vi "COD主界面（列队使用）.vi"() -> (8 "多列列表框":i32(listbox))   [LabVIEW 2016, in "斯坦道CODMn.lvlib"]
uses:
  <vilib>/Utility/miscctls.llb/LVPointTypeDef.ctl
  <vilib>/Plasmionique/MB Master/MB_Master_Serial/MB_Master_Serial.lvclass
  F:/Program Files/National Instruments/LabVIEW 2016/vi.lib/Plasmionique/MB Master/MB_Master/MB_Master.lvclass
  <vilib>/Plasmionique/MB Master/MB Master.lvlib
  <vilib>/ptbypt/NI_PtbyPt.lvlib
  PLC/PLC.lvlib
panel:
  out "启动选择 3":u16(ring) items=["COD水样测量", "COD标样核查", "COD零点核查", "COD加标回收", "COD平行样", "COD校零", "COD校标", ""]
  out "加热":bool
  out "搅拌":bool
  out "进硫酸":bool
  out "进草酸钠":bool
  out "进高锰酸钾":bool
  out "进加标回收样":bool
  out "进质控样":bool
  out "进标液":bool
  out "进蒸馏水":bool
  out "进水样":bool
  in  "定时启动":bool
  out "设置值":dbl
  out "系统时间":timestamp
  in  "时间校准":bool
  out "仪器时间":timestamp
  in  "修正系数 2":dbl
  in  "浓度 2":dbl
  in  "温度":dbl
  out "秒":u16
  out "分":u16
  in  "data in":T1
  out "数值":i32
  out "报警簇":T2
  out "读取参数":u16[](array[numeric])
  out "循环次数":i32
  out "DATABASE":u16[](array[numeric])
  out "Registers":u16[](array[numeric])
  in  "枚举":enum16{"读取数据", "写入数据", "读取写入DATABASE", "读取参数"}(ring)
  in  "Slave ID":u8=1
  in  "Serial Config":T3={"baud rate (bps)"=115200, "stop bits"=10, "parity"=0, "flow control"=0, "timeout"=1000, "retries"=1} {"stop bits" items=["1.0"=10, "1.5"=15, "2.0"=20]; "flow control" items=["None", "XON/XOFF", "RTS/CTS", "XON/XOFF & RTS/CTS", "DTR/DSR", "XON/XOFF & DTR/DSR"]; "parity" items=["None", "Odd", "Even", "Mark", "Space"]}
  out "COD浓度（mg/L)":dbl
  out "table 输入":string
  out "columns":string[](array[string])
  in  "保存":bool
  out "data":T4
  in  "温度 2":dbl
  in  "恒温时间":dbl
  in  "浓度":dbl
  in  "修正系数":dbl
  in  "基本量程":enum16{"10mL", "20mL"}(ring)
  in  "水样":dbl
  in  "蒸馏水":dbl
  in  "标液":dbl
  in  "质控样":dbl
  in  "加标回收":dbl
  in  "草酸钠":dbl
  in  "高锰酸钾":dbl
  in  "硫酸":dbl
  in  "关闭":bool
  in  "零点泵计量数 2":dbl
  in  "标度泵计量数 2":dbl
  in  "标样浓度 2":dbl
  out "进样管":dbl
  out "高锰酸钾":dbl
  out "草酸钠":dbl
  out "硫酸":dbl
  out "标度滴定值":dbl
  out "零点滴定值":dbl
  in  "启动":bool
  in  "故障清除":bool
  out "排液故障":bool
  out "进水样超量程":bool
  out "模式（受控）":u16
  out "ORP显示":dbl
  out "温度":dbl
  out "标样核查标记":bool
  out "平行样测量":bool
  out "加标回收测量":bool
  out "质控样测量":bool
  out "待机":bool
  out "校标错误":bool
  out "校零错误":bool
  out "测量错误":bool
  out "草酸钠报警":bool
  out "高锰酸钾报警":bool
  out "加热故障":bool
  out "温控器故障":bool
  out "ORP故障":bool
  out "排液标记":bool
  out "故障标记":bool
  out "校标标记":bool
  out "校零标记":bool
  out "通讯状态":bool
  out "水样测量":bool
  in  "参数配置":bool
  in  "VISA resource name":refnum<visa-resource-name>="COM3" caption="VISA资源名称"
  in  "停止":bool
  in  "单步启动":bool
  # "测量时间："
  # "水样~加标回收"
  # "mV"
  # "℃"
  # "注：遇到加热故障和排液故障时仪器不能正常启动，\n必须排查故障并点击报警清除按钮方可运行。"
  # "基本参数设置"
  # "泵计量参数设置"
  # "校零校标结果"
  # "加热恒温温度（℃）："
  # "水样："
  # "高锰酸钾："
  # "校零结果："
  # "校零滴定值："
  # "恒温时间（分钟）："
  # "蒸馏水："
  # "草酸钠："
  # "校标结果："
  # "标度滴定值："
  # "零点泵计量值："
  # "标准液浓度（mg/L）："
  # "标液："
  # "硫酸："
  # "标样浓度："
  # "标度泵计量值："
  # "修正系数："
  # "质控样："
  # "加标回收样："
  # "基本量程（20mL可选）："
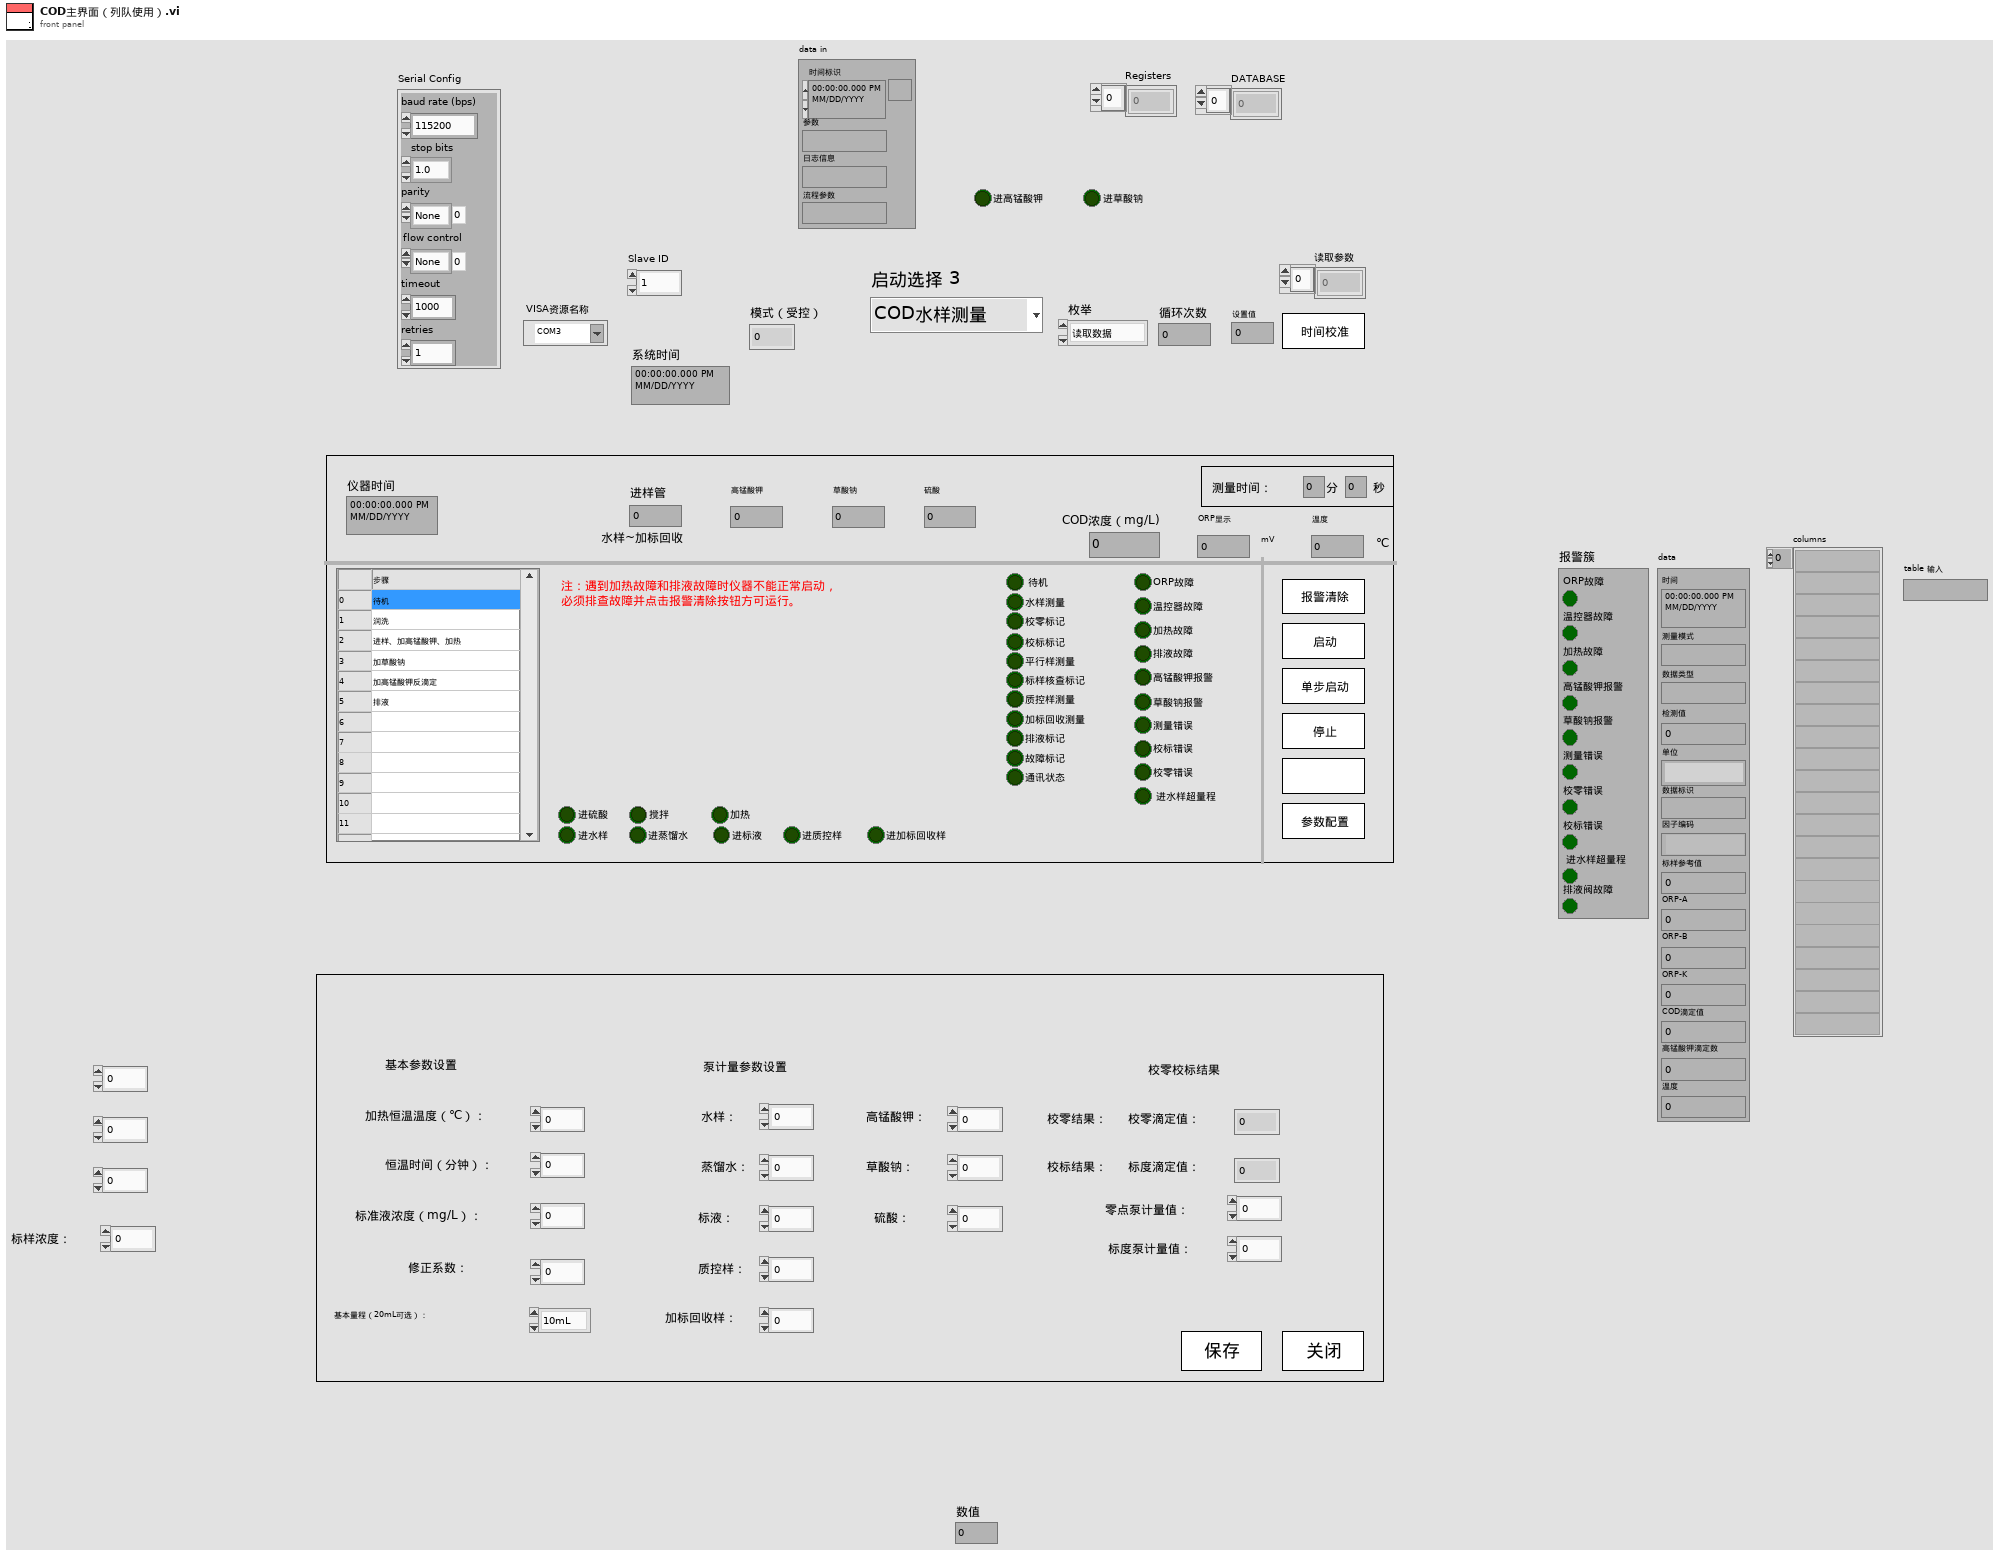
[diagram p1: front panel]
types:
  T1 = cluster{"时间标识":timestamp, "参数":string, "日志信息":string, "流程参数":string}
  T2 = cluster{"ORP故障":bool, "温控器故障":bool, "加热故障":bool, "高锰酸钾报警":bool, "草酸钠报警":bool, "测量错误":bool, "校零错误":bool, "校标错误":bool, " 进水样超量程":bool, "排液阀故障":bool}
  T3 = cluster{"baud rate (bps)":u32, "stop bits":u16, "parity":u16, "flow control":u16, "timeout":u32, "retries":i32}
  T4 = cluster{"时间":timestamp, "测量模式":string, "数据类型":string, "检测值":sgl, "单位":string, "数据标识":string, "因子编码":string, "标样参考值":sgl, "ORP-A":sgl, "ORP-B":sgl, "ORP-K":sgl, "COD滴定值":sgl, "高锰酸钾滴定数":sgl, "温度":sgl}
  T5 = cluster{"starting address":u16, "number of holding registers":u16}
  T6 = typedef "LVPointTypeDef.ctl" = cluster{"Horizontal":i16, "Vertical":i16}
  T7 = cluster{"测量模式":enum16{"水样测量", "标样核查", "零点核查", "加标回收", "平行样", "校零", "校标"}}
  T8 = cluster{"时间标识":timestamp, "设备":string, "日志信息":string}
  T9 = cluster{"时间标识":timestamp, "设备":string, "日志信息":string, "流程参数":string}
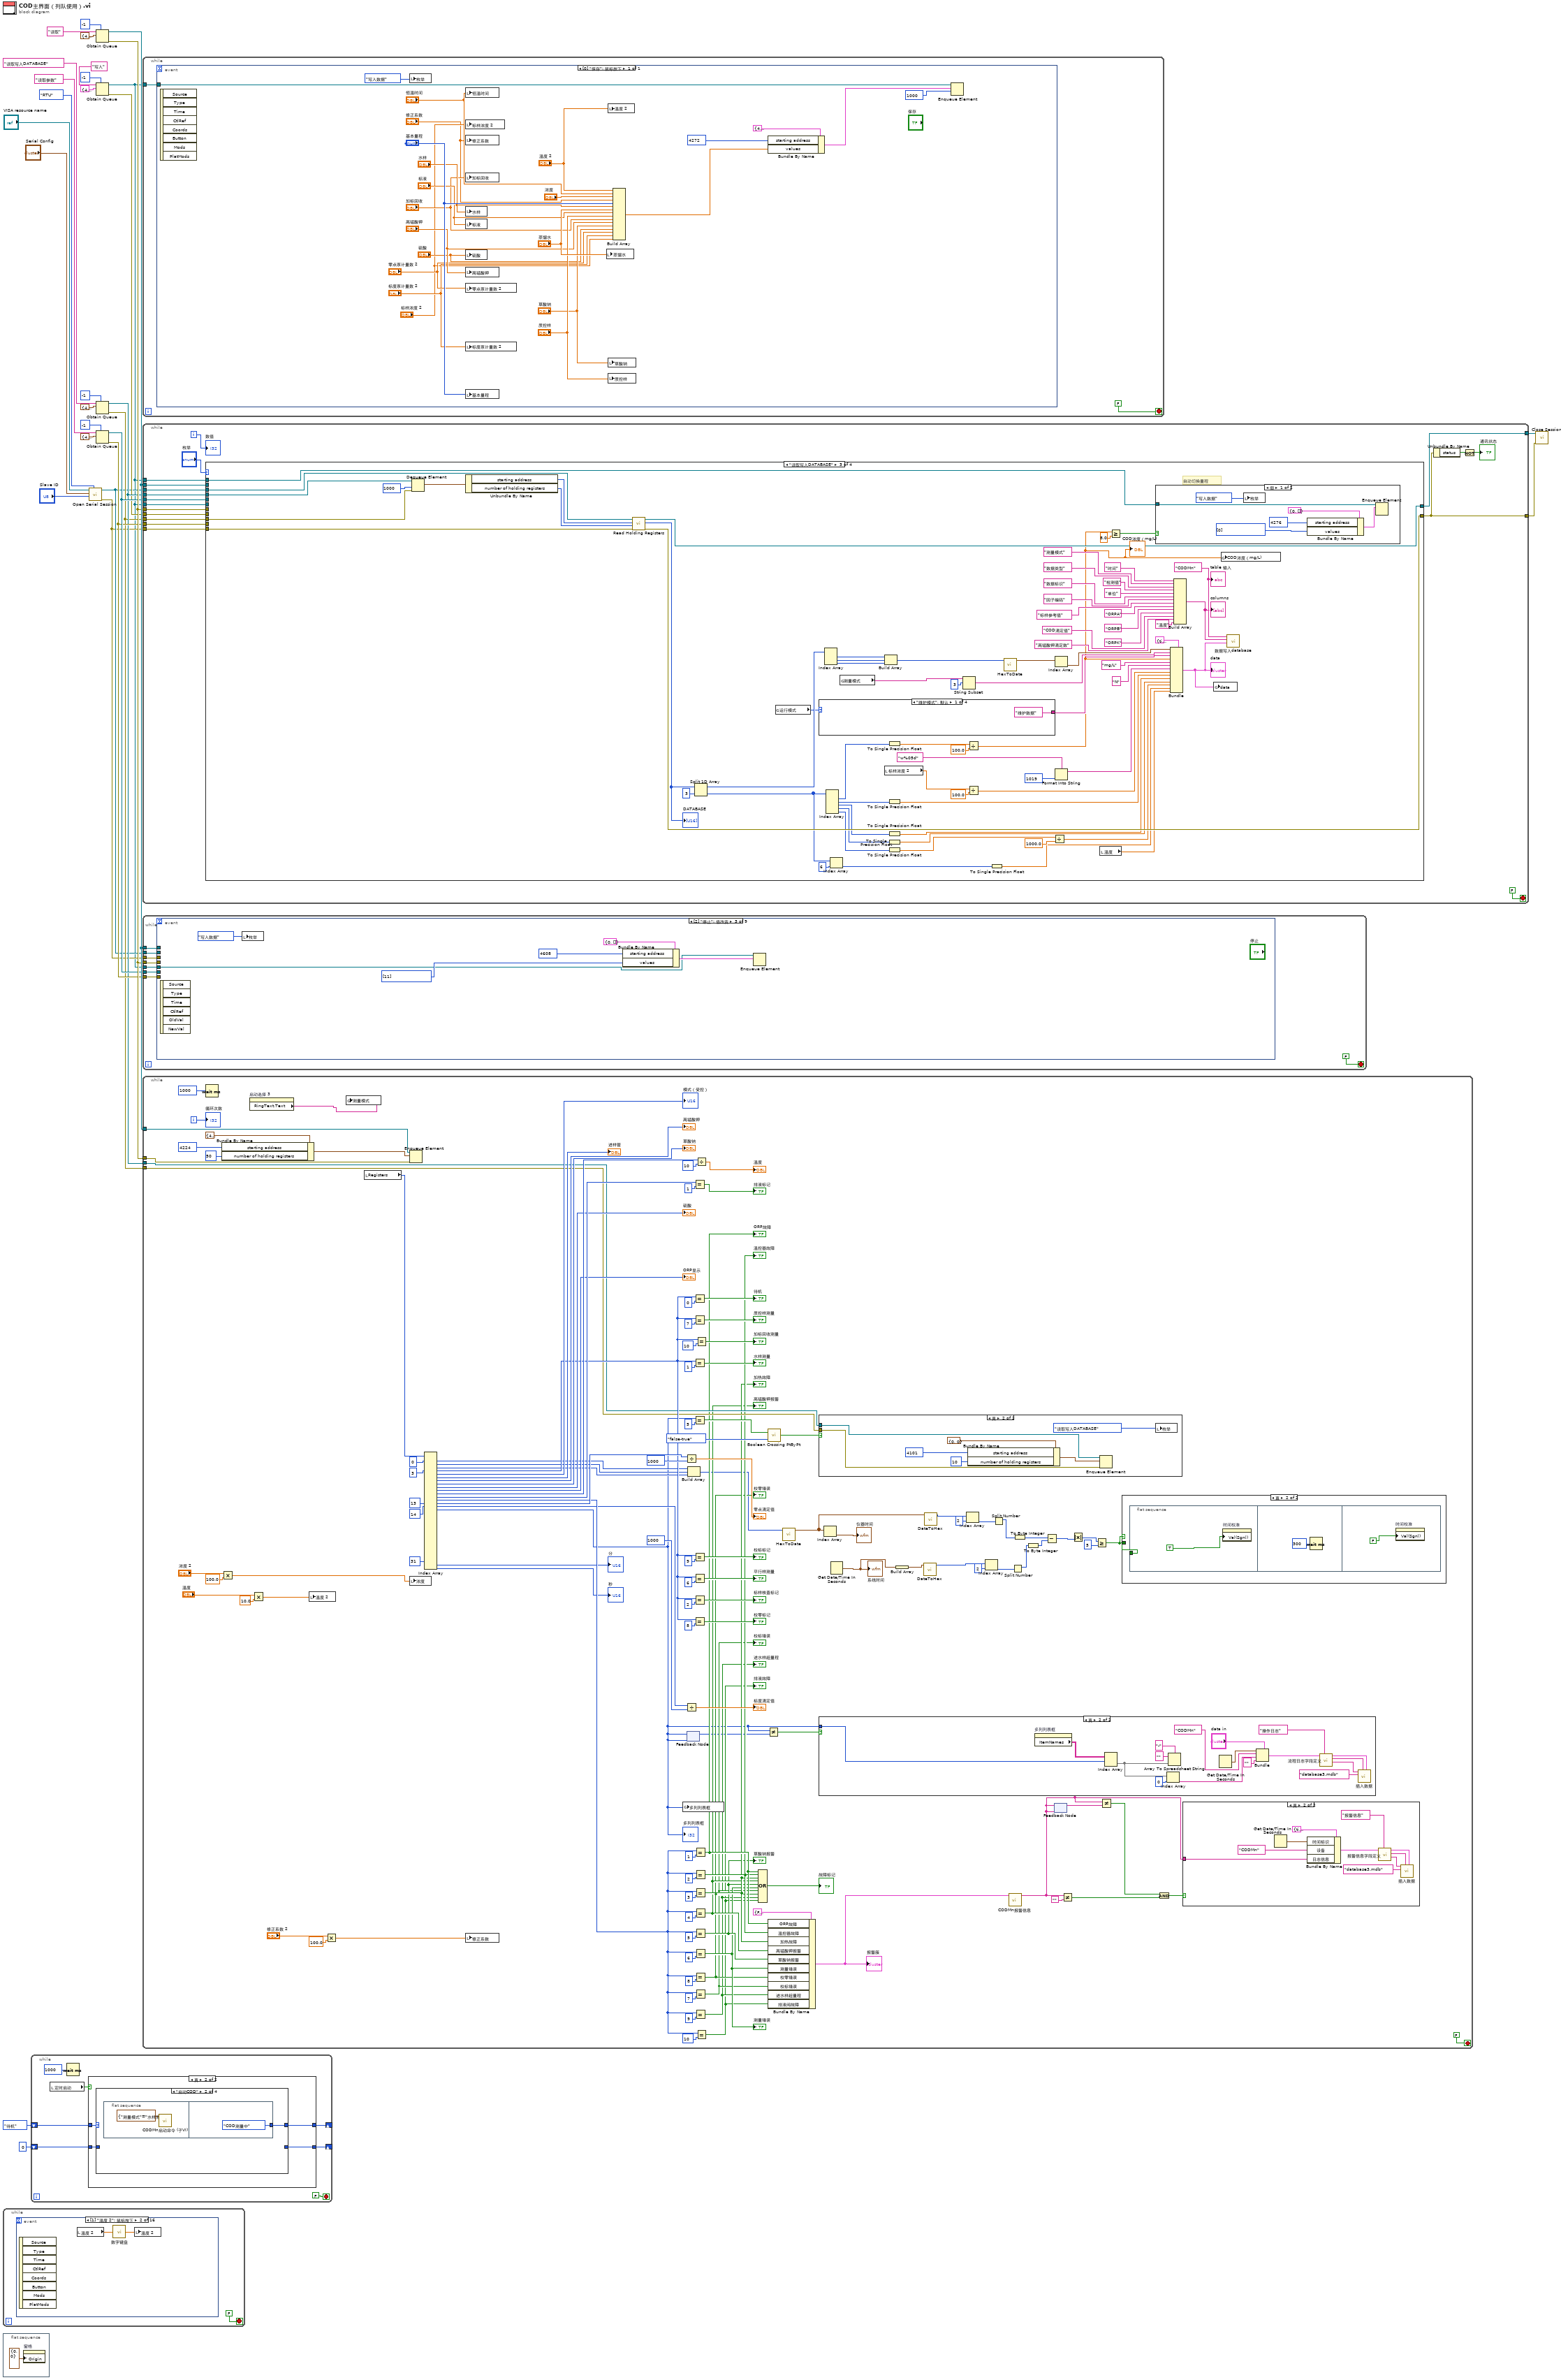
[diagram p0: block diagram]
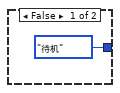
[diagram p2: hidden frame]
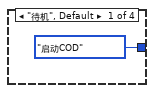
[diagram p3: hidden frame]
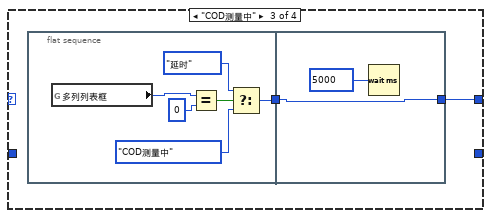
[diagram p4: hidden frame]
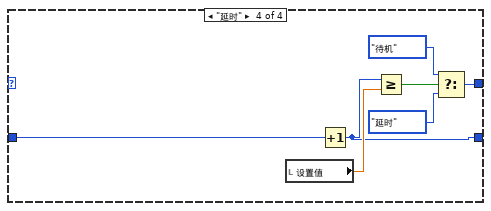
[diagram p5: hidden frame]
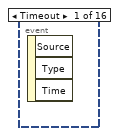
[diagram p10: hidden frame]
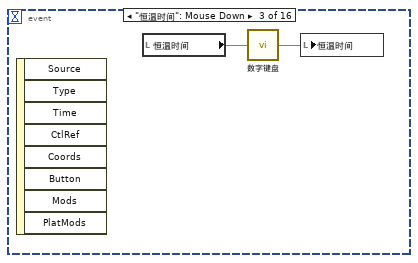
[diagram p11: hidden frame]
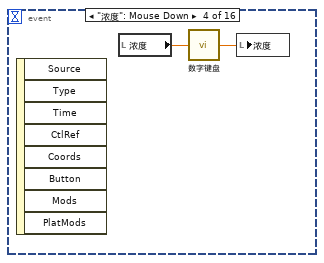
[diagram p12: hidden frame]
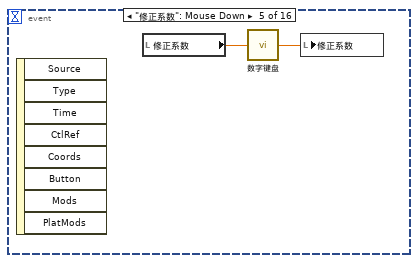
[diagram p13: hidden frame]
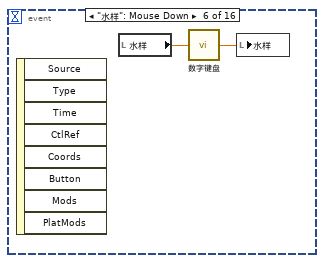
[diagram p14: hidden frame]
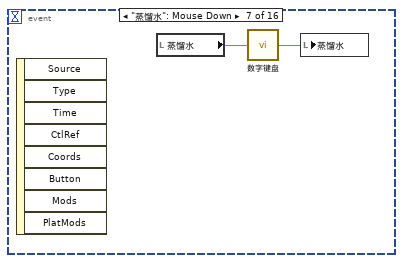
[diagram p15: hidden frame]
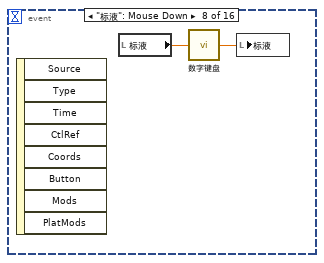
[diagram p16: hidden frame]
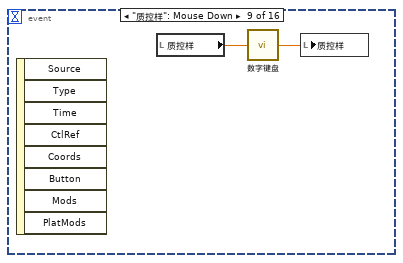
[diagram p17: hidden frame]
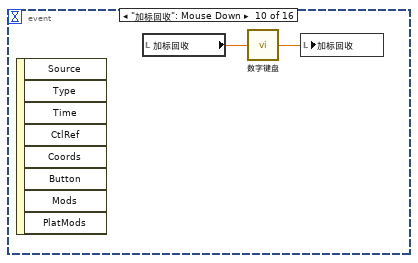
[diagram p18: hidden frame]
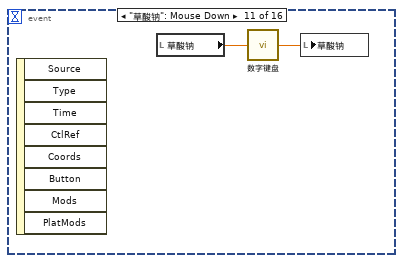
[diagram p19: hidden frame]
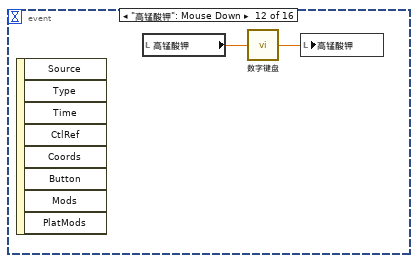
[diagram p20: hidden frame]
diagram:
  n1 = while {
    stop <- FALSE stop-if-true
    n2 = event shown="[1] \"温度 2\": 鼠标按下" {
      selector: _ -> [_ _ _ _ _ _ _ _ _ _ _ _ _ _ _ _]
      dyn-events: _ -> [_ _ _ _ _ _ _ _ _ _ _ _ _ _ _ _]
      timeout: _ -> [_ _ _ _ _ _ _ _ _ _ _ _ _ _ _ _]
      event Timeout {
        n3 = event-data() -> ()  [unwired: 1 in, 3 out]
      }
      event "温度 2": Mouse Down {
        n4 = event-data() -> ()  [unwired: 1 in, 8 out]
        n5 = local read "温度 2"() -> (w32:dbl)
        n6 = call "数字键盘.vi"("OldNumber"=w32) -> ("NewNumber"=w33:sgl)
        n7 = local write "温度 2"(w33) -> ()
      }
      event "恒温时间": Mouse Down {
        n8 = event-data() -> ()  [unwired: 1 in, 8 out]
        n9 = local read "恒温时间"() -> (w34:dbl)
        n10 = call "数字键盘.vi"("OldNumber"=w34) -> ("NewNumber"=w35:sgl)
        n11 = local write "恒温时间"(w35) -> ()
      }
      event "浓度": Mouse Down {
        n12 = event-data() -> ()  [unwired: 1 in, 8 out]
        n13 = local read "浓度"() -> (w36:dbl)
        n14 = call "数字键盘.vi"("OldNumber"=w36) -> ("NewNumber"=w37:sgl)
        n15 = local write "浓度"(w37) -> ()
      }
      event "修正系数": Mouse Down {
        n16 = event-data() -> ()  [unwired: 1 in, 8 out]
        n17 = local read "修正系数"() -> (w38:dbl)
        n18 = call "数字键盘.vi"("OldNumber"=w38) -> ("NewNumber"=w39:sgl)
        n19 = local write "修正系数"(w39) -> ()
      }
      event "水样": Mouse Down {
        n20 = event-data() -> ()  [unwired: 1 in, 8 out]
        n21 = local read "水样"() -> (w40:dbl)
        n22 = call "数字键盘.vi"("OldNumber"=w40) -> ("NewNumber"=w41:sgl)
        n23 = local write "水样"(w41) -> ()
      }
      event "蒸馏水": Mouse Down {
        n24 = event-data() -> ()  [unwired: 1 in, 8 out]
        n25 = local read "蒸馏水"() -> (w42:dbl)
        n26 = call "数字键盘.vi"("OldNumber"=w42) -> ("NewNumber"=w43:sgl)
        n27 = local write "蒸馏水"(w43) -> ()
      }
      event "标液": Mouse Down {
        n28 = event-data() -> ()  [unwired: 1 in, 8 out]
        n29 = local read "标液"() -> (w44:dbl)
        n30 = call "数字键盘.vi"("OldNumber"=w44) -> ("NewNumber"=w45:sgl)
        n31 = local write "标液"(w45) -> ()
      }
      event "质控样": Mouse Down {
        n32 = event-data() -> ()  [unwired: 1 in, 8 out]
        n33 = local read "质控样"() -> (w46:dbl)
        n34 = call "数字键盘.vi"("OldNumber"=w46) -> ("NewNumber"=w47:sgl)
        n35 = local write "质控样"(w47) -> ()
      }
      event "加标回收": Mouse Down {
        n36 = event-data() -> ()  [unwired: 1 in, 8 out]
        n37 = local read "加标回收"() -> (w48:dbl)
        n38 = call "数字键盘.vi"("OldNumber"=w48) -> ("NewNumber"=w49:sgl)
        n39 = local write "加标回收"(w49) -> ()
      }
      event "草酸钠": Mouse Down {
        n40 = event-data() -> ()  [unwired: 1 in, 8 out]
        n41 = local read "草酸钠"() -> (w50:dbl)
        n42 = call "数字键盘.vi"("OldNumber"=w50) -> ("NewNumber"=w51:sgl)
        n43 = local write "草酸钠"(w51) -> ()
      }
      event "高锰酸钾": Mouse Down {
        n44 = event-data() -> ()  [unwired: 1 in, 8 out]
        n45 = local read "高锰酸钾"() -> (w52:dbl)
        n46 = call "数字键盘.vi"("OldNumber"=w52) -> ("NewNumber"=w53:sgl)
        n47 = local write "高锰酸钾"(w53) -> ()
      }
      event "硫酸": Mouse Down {
        n48 = event-data() -> ()  [unwired: 1 in, 8 out]
        n49 = local read "硫酸"() -> (w54:dbl)
        n50 = call "数字键盘.vi"("OldNumber"=w54) -> ("NewNumber"=w55:sgl)
        n51 = local write "硫酸"(w55) -> ()
      }
      event "零点泵计量数 2": Mouse Down {
        n52 = event-data() -> ()  [unwired: 1 in, 8 out]
        n53 = local read "零点泵计量数 2"() -> (w56:dbl)
        n54 = call "数字键盘.vi"("OldNumber"=w56) -> ("NewNumber"=w57:sgl)
        n55 = local write "零点泵计量数 2"(w57) -> ()
      }
      event "标度泵计量数 2": Mouse Down {
        n56 = event-data() -> ()  [unwired: 1 in, 8 out]
        n57 = local read "标度泵计量数 2"() -> (w58:dbl)
        n58 = call "数字键盘.vi"("OldNumber"=w58) -> ("NewNumber"=w59:sgl)
        n59 = local write "标度泵计量数 2"(w59) -> ()
      }
      event "标样浓度 2": Mouse Down {
        n60 = event-data() -> ()  [unwired: 1 in, 8 out]
        n61 = local read "标样浓度 2"() -> (w60:dbl)
        n62 = call "数字键盘.vi"("OldNumber"=w60) -> ("NewNumber"=w61:sgl)
        n63 = local write "标样浓度 2"(w61) -> ()
      }
    }
  }
  n64 = flat-sequence {
    frame #0 {
      n65 = property on="窗格" class="Pane"("Origin"=T6 {"Horizontal"=0, "Vertical"=0} ("原点")) -> ()  [unwired: 2 in, 2 out]
    }
  }
  n66 = while {
    shift-right: [w64] -> _
    shift-left: enum16{"待机", "启动COD", "COD测量中", "延时"}."待机" -> [w66]
    shift-right: [w63] -> _
    shift-left: 0 -> [w65]
    stop <- FALSE stop-if-true
    n67 = local read "定时启动"() -> (w68:bool)
    n68 = Wait (ms)(milliseconds to wait=u32 1000 ("等待时间（毫秒）")) -> ()  [unwired: 1 out]
    n69 = case shown="真" w68 {
      tunnel: w66 -> [_ w74]
      tunnel: w65 -> [_ w73]
      tunnel: [enum16{"待机", "启动COD", "COD测量中", "延时"}."待机" w72] -> w64
      tunnel: [_ w71] -> w63
      frame False {
      }
      frame True {
        n70 = case shown="\"启动COD\"" w74 {
          tunnel: w73 -> [_ _ _ w95]
          tunnel: [enum16{"待机", "启动COD", "COD测量中", "延时"}."启动COD" w76 w80 w89] -> w72
          tunnel: [_ _ _ w92] -> w71
          frame "待机", Default {
          }
          frame "启动COD" {
            n71 = flat-sequence {
              tunnel: [enum16{"待机", "启动COD", "COD测量中", "延时"}."COD测量中"] -> w76
              frame #0 {
                n72 = call "CODMn启动命令 (子VI).vi"("启动测量模式"=T7 {"测量模式"=enum."水样测量"}) -> ()  [unwired: 11 in]
              }
              frame #1 {
              }
            }
          }
          frame "COD测量中" {
            n73 = flat-sequence {
              tunnel: [w81] -> w79
              tunnel: [w88] -> w80
              tunnel: w79 -> [w88]
              frame #0 {
                n74 = global read "运行时序全局变量.vi" "多列列表框"() -> (w86:i32)
                n75 = Equal?(x=w86, y=0) -> (x = y?=w84:bool)
                n76 = Select(t=enum16{"待机", "启动COD", "COD测量中", "延时"}."延时", s=w84, f=enum16{"待机", "启动COD", "COD测量中", "延时"}."COD测量中") -> (s? t:f=w81:enum16{"待机", "启动COD", "COD测量中", "延时"})
              }
              frame #1 {
                n77 = Wait (ms)(milliseconds to wait=u32 5000 ("等待时间（毫秒）")) -> ()  [unwired: 1 out]
              }
            }
          }
          frame "延时" {
            n78 = local read "设置值"() -> (w94:dbl)
            n79 = Increment(x=w95) -> (x+1=w92:i32)
            n80 = Greater Or Equal?(x=w92, y=w94) -> (x >= y?=w93:bool)
            n81 = Select(t=enum16{"待机", "启动COD", "COD测量中", "延时"}."待机", s=w93, f=enum16{"待机", "启动COD", "COD测量中", "延时"}."延时") -> (s? t:f=w89:enum16{"待机", "启动COD", "COD测量中", "延时"})
          }
        }
      }
    }
  }
  n82 = call <vilib>:"Open Serial Session.vi"("Mode (RTU)"=enum16{"RTU", "ASCII"}."RTU", "Slave ID"="Slave ID", "Serial Config"="Serial Config", "VISA Resource"="VISA resource name") -> ("Error out"=w4:errorcluster, "MB_Serial session"=w5:refnum<class "MB_Master_Serial.lvclass">)  [unwired: 6 in]
  n83 = Obtain Queue(max queue size (-1, unlimited)=-1 ("队列最大值（-1，无限）"), name (unnamed)="读取" ("名称（未命名）"), element data type=T5 {"starting address"=4224, "number of holding registers"=16}) -> (queue out=w20:refnum<queue>, error out=w19:errorcluster)  [unwired: 2 in, 1 out]
  n84 = Obtain Queue(max queue size (-1, unlimited)=-1 ("队列最大值（-1，无限）"), name (unnamed)="写入" ("名称（未命名）"), element data type=cluster{"starting address":u16, "values":u16[]} {"starting address"=4272, "values"=[]}) -> (queue out=w1:refnum<queue>, error out=w6:errorcluster)  [unwired: 2 in, 1 out]
  n85 = Obtain Queue(max queue size (-1, unlimited)=-1 ("队列最大值（-1，无限）"), name (unnamed)="读取写入DATABASE" ("名称（未命名）"), element data type=T5 {"starting address"=4224, "number of holding registers"=16}) -> (queue out=w8:refnum<queue>, error out=w7:errorcluster)  [unwired: 2 in, 1 out]
  n86 = Obtain Queue(max queue size (-1, unlimited)=-1 ("队列最大值（-1，无限）"), name (unnamed)="读取参数" ("名称（未命名）"), element data type=T5 {"starting address"=4224, "number of holding registers"=16}) -> (queue out=w13:refnum<queue>, error out=w12:errorcluster)  [unwired: 2 in, 1 out]
  n87 = while {
    tunnel: w1 -> [w97]
    stop <- FALSE stop-if-true
    n88 = event shown="[0] \"保存\": 鼠标按下" {
      selector: _ -> [_]
      dyn-events: _ -> [_]
      timeout: _ -> [_]
      tunnel: w97 -> [w107]
      event "保存": Mouse Down {
        n89 = event-data() -> ()  [unwired: 1 in, 8 out]
        n90 = local write "枚举"(enum16{"读取数据", "写入数据", "读取写入DATABASE", "读取参数"}."写入数据" ("枚举")) -> ()
        n91 = local write "恒温时间"("恒温时间") -> ()
        n92 = local write "标样浓度 2"("标样浓度 2") -> ()
        n93 = local write "修正系数"("修正系数") -> ()
        n94 = local write "加标回收"("加标回收") -> ()
        n95 = local write "水样"("水样") -> ()
        n96 = local write "标液"("标液") -> ()
        n97 = local write "硫酸"("硫酸") -> ()
        n98 = local write "高锰酸钾"("高锰酸钾") -> ()
        n99 = local write "零点泵计量数 2"("零点泵计量数 2") -> ()
        n100 = local write "标度泵计量数 2"("标度泵计量数 2") -> ()
        n101 = local write "基本量程"("基本量程") -> ()
        n102 = local write "蒸馏水"("蒸馏水") -> ()
        n103 = local write "温度 2"("温度 2") -> ()
        n104 = local write "草酸钠"("草酸钠") -> ()
        n105 = local write "质控样"("质控样") -> ()
        n106 = Build Array("温度 2", "恒温时间", "浓度", "修正系数", "基本量程", "水样", "蒸馏水", "标液", "质控样", "加标回收", "高锰酸钾", "草酸钠", "硫酸", "零点泵计量数 2", "标度泵计量数 2", "标样浓度 2") -> (w105:dbl[])
        n107 = Bundle By Name(cluster=cluster{"starting address":u16, "values":u16[]} {"starting address"=4272, "values"=[]}, "starting address"=u16 4272, "values"=w105) -> (w103:cluster{"starting address":u16, "values":u16[]})
        n108 = Enqueue Element(queue=w107, element=w103, timeout in ms (-1)=1000 ("超时毫秒(-1)")) -> ()  [unwired: 1 in, 3 out]
      }
    }
  }
  n109 = while {
    tunnel: w5 -> [w138]
    tunnel: w4 -> [w137]
    tunnel: w1 -> [w136]
    tunnel: w20 -> [w135]
    tunnel: w19 -> [w134]
    tunnel: [w124] -> w18
    tunnel: [w133] -> w17
    tunnel: w13 -> [w131]
    tunnel: w12 -> [w130]
    tunnel: w8 -> [w129]
    tunnel: w7 -> [w128]
    tunnel: w6 -> [w127]
    tunnel: w1 -> [w121]
    i -> [w123]
    stop <- FALSE stop-if-true
    n110 = case shown="\"读取写入DATABASE\"" "枚举" {
      tunnel: w138 -> [w174 w182 w262 w311]
      tunnel: w137 -> [w173 w178 w261 w310]
      tunnel: w136 -> [_ w181 _ _]
      tunnel: [w147 w180 w264 w313] -> w133
      tunnel: [w146 w179 w263 w312] -> w124
      tunnel: w135 -> [w171 _ _ _]
      tunnel: w134 -> [w167 _ _ _]
      tunnel: w131 -> [_ _ _ w309]
      tunnel: w130 -> [_ _ _ w308]
      tunnel: w129 -> [_ _ w260 _]
      tunnel: w128 -> [_ _ w259 _]
      tunnel: w127 -> [_ w177 _ _]
      tunnel: w121 -> [_ _ w199 _]
      frame "读取数据", Default {
        n111 = Dequeue Element(queue=w171, timeout in ms (-1)=1000 ("超时毫秒(-1)"), error in (no error)=w167) -> (element=w170:T5)  [unwired: 3 out]
        n112 = Unbundle By Name(w170) -> ("starting address"=w169:u16, "number of holding registers"=w168:u16)
        n113 = call <vilib>:"Read Holding Registers.vi"("error in (no error)"=w173, "quantity"=w168, "starting address"=w169, "MB session in"=w174) -> ("error out"=w162:errorcluster, "Registers"=→"Registers":u16[], "MB session out"=w165:refnum<class "MB_Master_Serial.lvclass">)  [unwired: 5 in]
        n114 = call <vilib>:"Read Coils.vi"("error in (no error)"=w162, "quantity"=u16 8, "starting address"=u16 140, "MB session in"=w165) -> ("error out"=w152:errorcluster, "Coils"=w161:bool[], "MB session out"=w153:refnum<class "MB_Master_Serial.lvclass">)  [unwired: 5 in]
        n115 = Index Array(array=w161) -> (element #1=→"进水样":bool, element #2=→"进蒸馏水":bool, element #3=→"进标液":bool, element #4=→"进质控样":bool, element #5=→"进加标回收样":bool, element #6=→"进高锰酸钾":bool, element #7=→"进草酸钠":bool, element #8=→"进硫酸":bool)  [unwired: 9 in, 1 out]
        n116 = call <vilib>:"Read Coils.vi"("error in (no error)"=w152, "quantity"=u16 1, "starting address"=u16 137, "MB session in"=w153) -> ("error out"=w148:errorcluster, "Coils"=w140:bool[], "MB session out"=w149:refnum<class "MB_Master_Serial.lvclass">)  [unwired: 5 in]
        n117 = Index Array(array=w140) -> (element=→"搅拌":bool)  [unwired: 1 in]
        n118 = call <vilib>:"Read Coils.vi"("error in (no error)"=w148, "quantity"=u16 1, "starting address"=u16 400, "MB session in"=w149) -> ("error out"=w146:errorcluster, "Coils"=w143:bool[], "MB session out"=w147:refnum<class "MB_Master_Serial.lvclass">)  [unwired: 5 in]
        n119 = Index Array(array=w143) -> (element=→"加热":bool)  [unwired: 1 in]
      }
      frame "写入数据" {
        n120 = flat-sequence {
          tunnel: w182 -> [w192]
          tunnel: w181 -> [w191]
          tunnel: w178 -> [w185]
          tunnel: w177 -> [w184]
          tunnel: [w187] -> w176
          tunnel: [w186] -> w175
          tunnel: [w194] -> w179
          tunnel: [w195] -> w180
          tunnel: w176 -> [w195]
          tunnel: w175 -> [w194]
          frame #0 {
            n121 = Dequeue Element(queue=w191, error in (no error)=w184) -> (queue out=w183:refnum<queue>, element=w190:cluster{"starting address":u16, "values":u16[]})  [unwired: 1 in, 2 out]
            n122 = Flush Queue(queue=w183) -> ()  [unwired: 1 in, 3 out]
            n123 = Unbundle By Name(w190) -> ("starting address"=w189:u16, "values"=w188:u16[])
            n124 = call <vilib>:"Write Multiple Registers.vi"("error in (no error)"=w185, "values"=w188, "starting address"=w189, "MB session in"=w192) -> ("error out"=w186:errorcluster, "MB session out"=w187:refnum<class "MB_Master_Serial.lvclass">)  [unwired: 6 in]
          }
          frame #1 {
            n125 = local write "枚举"(enum16{"读取数据", "写入数据", "读取写入DATABASE", "读取参数"}."读取数据" ("枚举")) -> ()
          }
        }
      }
      frame "读取写入DATABASE" {
        w227 = "CODMn" ("table")
        # "自动切换量程"
        n126 = Dequeue Element(queue=w260, timeout in ms (-1)=1000 ("超时毫秒(-1)"), error in (no error)=w259) -> (element=w267:T5)  [unwired: 3 out]
        n127 = Unbundle By Name(w267) -> ("starting address"=w266:u16, "number of holding registers"=w265:u16)
        n128 = call <vilib>:"Read Holding Registers.vi"("error in (no error)"=w261, "quantity"=w265, "starting address"=w266, "MB session in"=w262) -> ("error out"=w263:errorcluster, "Registers"=w223:u16[], "MB session out"=w264:refnum<class "MB_Master_Serial.lvclass">)  [unwired: 5 in]
        "DATABASE" <- w223
        n129 = Split 1D Array(array=w223, index=3 ("索引")) -> (first subarray=w257:u16[], second subarray=w245:u16[])
        n130 = global read "系统变量.vi" "运行模式"() -> (w206:enum16{"维护模式", "常规模式", "应急模式", "质控模式"})
        n131 = case shown="\"维护模式\", 默认" w206 {
          tunnel: ["维护数据" ("单位") "常规数据" ("单位") "常规数据" ("单位") "常规数据" ("单位")] -> w205
          frame "维护模式", Default {
          }
          frame "常规模式" {
          }
          frame "应急模式" {
          }
          frame "质控模式" {
          }
        }
        n132 = Index Array(array=w257) -> (element #1=w255:u16, element #2=w254:u16, element #3=w253:u16)  [unwired: 3 in]
        n133 = Index Array(array=w245) -> (element #1=w250:u16, element #2=w249:u16, element #3=w248:u16, element #4=w247:u16, element #5=w246:u16)  [unwired: 5 in]
        n134 = Index Array(array=w245, index=6 ("索引")) -> (element=w243:u16)
        n135 = global read "COD测量模式全局.vi" "测量模式"() -> (w196:string)
        n136 = Build Array(w255, w254, w253) -> (w252:u16[])
        n137 = local read "标样浓度 2"() -> (w221:dbl)
        n138 = To Single Precision Float(number=w250) -> (single precision float=w242:sgl)
        n139 = To Single Precision Float(number=w249) -> (single precision float=w211:sgl)
        n140 = To Single Precision Float(number=w248) -> (single precision float=w212:sgl)
        n141 = To Single Precision Float(number=w247) -> (single precision float=w213:sgl)
        n142 = To Single Precision Float(number=w246) -> (single precision float=w239:sgl)
        n143 = String Subset(string=w196, offset (0)=3 ("偏移量(0)")) -> (substring=w202:string)  [unwired: 1 in]
        n144 = Divide(x=w242, y=sgl 100.0) -> (x/y=w197:sgl)
        "COD浓度（mg/L)" <- w197
        n145 = Divide(x=w221, y=100.0) -> (x/y=w210:dbl)
        n146 = To Single Precision Float(number=w243) -> (single precision float=w215:sgl)
        n147 = call "HexToDate.vi"("数组"=w252) -> ("DATE"=w256:timestamp[])  [unwired: 10 in]
        n148 = Divide(x=w239, y=sgl 1000.0) -> (x/y=w214:sgl)
        n149 = Index Array(array=w256) -> (element=w251:timestamp)  [unwired: 1 in]
        n150 = Format Into String(format string="w%05d" ("格式字符串"), u32 1019 ("因子编码")) -> (resulting string=w209:string)  [unwired: 2 in, 1 out]
        n151 = local read "温度"() -> (w204:dbl)
        n152 = Greater Or Equal?(x=w197, y=sgl 8.0) -> (x >= y?=w200:bool)
        n153 = case shown="假" w200 {
          tunnel: w199 -> [w268 w277]
          frame False {
            n154 = local write "枚举"(enum16{"读取数据", "写入数据", "读取写入DATABASE", "读取参数"}."写入数据" ("枚举")) -> ()
            n155 = Bundle By Name(cluster=cluster{"starting address":u16, "values":u16[]} {"starting address"=0, "values"=[]}, "starting address"=u16 4276, "values"=u16[] [0]) -> (w271:cluster{"starting address":u16, "values":u16[]})
            n156 = Enqueue Element(queue=w268, element=w271) -> ()  [unwired: 2 in, 3 out]
          }
          frame True {
            n157 = local write "枚举"(enum16{"读取数据", "写入数据", "读取写入DATABASE", "读取参数"}."写入数据" ("枚举")) -> ()
            n158 = Bundle By Name(cluster=cluster{"starting address":u16, "values":u16[]} {"starting address"=0, "values"=[]}, "starting address"=u16 4276, "values"=u16[] [1]) -> (w278:cluster{"starting address":u16, "values":u16[]})
            n159 = Enqueue Element(queue=w277, element=w278) -> ()  [unwired: 2 in, 3 out]
          }
        }
        n160 = Bundle(cluster=T4 {"时间"=timestamp(0 s since 1904-01-01), "测量模式"="", "数据类型"="", "检测值"=0.0, "单位"="", "数据标识"="", "因子编码"="", "标样参考值"=0.0, "ORP-A"=0.0, "ORP-B"=0.0, "ORP-K"=0.0, "COD滴定值"=0.0, "高锰酸钾滴定数"=0.0, "温度"=0.0} ("data"), "时间"=w251, "测量模式"=w202, "数据类型"=w205, "检测值"=w197, "单位"="mg/L", "数据标识"="N", "因子编码"=w209, "标样参考值"=w210, "ORP-A"=w211, "ORP-B"=w212, "ORP-K"=w213, "COD滴定值"=w214, "高锰酸钾滴定数"=w215, "温度"=w204) -> (w198:T4)
        "data" <- w198
        n161 = Build Array("时间", "测量模式", "数据类型", "检测值", "单位", "数据标识", "因子编码", "标样参考值", "ORPA", "ORPB", "ORPK", "COD滴定值", "高锰酸钾滴定数", "温度") -> (w226:string[])
        "columns" <- w226
        n162 = global write "COD读取DATA全局.vi" "data"(w198) -> ()
        n163 = global write "COD浓度全局变量.vi" "COD浓度（mg/L)"(w197) -> ()
        n164 = call "数据写入database.vi"("data"=w198, "columns"=w226, "table"=w227) -> ()  [unwired: 9 in]
        "table 输入" <- w227
      }
      frame "读取参数" {
        n165 = Dequeue Element(queue=w309, timeout in ms (-1)=1000 ("超时毫秒(-1)"), error in (no error)=w308) -> (element=w317:T5)  [unwired: 3 out]
        n166 = local write "枚举"(enum16{"读取数据", "写入数据", "读取写入DATABASE", "读取参数"}."读取数据" ("枚举")) -> ()
        n167 = Unbundle By Name(w317) -> ("starting address"=w316:u16, "number of holding registers"=w315:u16)
        n168 = call <vilib>:"Read Holding Registers.vi"("error in (no error)"=w310, "quantity"=w315, "starting address"=w316, "MB session in"=w311) -> ("error out"=w312:errorcluster, "Registers"=w294:u16[], "MB session out"=w313:refnum<class "MB_Master_Serial.lvclass">)  [unwired: 5 in]
        "读取参数" <- w294
        n169 = Index Array(array=w294) -> (element #1=w287:u16, element #2=w307:u16, element #3=w306:u16, element #4=w285:u16, element #5=w305:u16, element #6=w304:u16, element #7=w303:u16, element #8=w302:u16, element #9=w301:u16, element #10=w300:u16, element #11=w299:u16, element #12=w298:u16, element #13=w297:u16, element #14=w296:u16, element #15=w295:u16, element #16=w292:u16)  [unwired: 16 in]
        n170 = local write "浓度"(w306) -> ()
        n171 = local write "水样"(w304) -> ()
        n172 = local write "硫酸"(w297) -> ()
        n173 = local write "标液"(w302) -> ()
        n174 = local write "恒温时间"(w307) -> ()
        n175 = local write "基本量程"(w305) -> ()
        n176 = local write "加标回收"(w300) -> ()
        n177 = local write "高锰酸钾"(w299) -> ()
        n178 = local write "草酸钠"(w298) -> ()
        n179 = local write "零点泵计量数 2"(w296) -> ()
        n180 = local write "标度泵计量数 2"(w295) -> ()
        n181 = local write "蒸馏水"(w303) -> ()
        n182 = local write "质控样"(w301) -> ()
        n183 = Divide(x=w287, y=u16 10) -> (x/y=w288:dbl)
        n184 = Divide(x=w285, y=u16 100) -> (x/y=w284:dbl)
        n185 = Divide(x=w292, y=u16 100) -> (x/y=w291:dbl)
        n186 = local write "温度"(w288) -> ()
        n187 = local write "修正系数 2"(w284) -> ()
        n188 = local write "浓度 2"(w291) -> ()
      }
    }
    n189 = Unbundle By Name(w124) -> ("status"=w125:bool)
    n190 = Not(x=w125) -> (.not. x?=→"通讯状态":bool)
    "数值" <- w123
  }
  n191 = while {
    tunnel: w20 -> [w325]
    tunnel: w19 -> [w324]
    tunnel: w1 -> [w323]
    tunnel: w13 -> [w322]
    tunnel: w12 -> [w321]
    tunnel: w5 -> [w319]
    tunnel: w4 -> [w318]
    stop <- FALSE stop-if-true
    n192 = event shown="[2] \"停止\": 值改变" {
      selector: _ -> [_ _ _ _ _ _ _ _ _]
      dyn-events: _ -> [_ _ _ _ _ _ _ _ _]
      timeout: _ -> [_ _ _ _ _ _ _ _ _]
      tunnel: w325 -> [_ _ _ _ _ _ _ _ _]
      tunnel: w324 -> [_ _ _ _ _ _ _ _ _]
      tunnel: w323 -> [w332 w366 w387 _ _ _ w405 w419 _]
      tunnel: w322 -> [_ _ _ w393 _ _ _ _ _]
      tunnel: w321 -> [_ _ _ w392 _ _ _ _ _]
      tunnel: w319 -> [_ _ _ _ _ w404 _ _ _]
      tunnel: w318 -> [_ _ _ _ _ w403 _ _ _]
      event "单步启动": Mouse Down {
        n193 = event-data() -> ()  [unwired: 1 in, 8 out]
        n194 = call "单步启动选择对话框.vi"() -> ("启动选择 2"=w335:u16)  [unwired: 10 in, 1 out]
        n195 = case shown="0" w335 {
          tunnel: [u16 4610 ("address") u16 4610 ("address") u16 4610 ("address") u16 4610 ("address") u16 4610 ("address") u16 4610 ("address") u16 4610 ("address") u16 4610 ("address") u16 4610 ("address") u16 4610 ("address") u16 4610 ("address") u16 4610 ("address")] -> w331
          tunnel: [u16 1 ("address") u16 2 ("address") u16 3 ("address") u16 4 ("address") u16 5 ("address") u16 6 ("address") u16 7 ("address") u16 8 ("address") u16 9 ("holding register value") u16 10 ("holding register value") u16 11 ("holding register value") u16 0 ("address")] -> w328
          frame 0 {
          }
          frame 1 {
          }
          frame 2 {
          }
          frame 3 {
          }
          frame 4 {
          }
          frame 5 {
          }
          frame 6 {
          }
          frame 7 {
          }
          frame 8 {
          }
          frame 9 {
          }
          frame 10 {
          }
          frame 11, Default {
          }
        }
        n196 = local write "枚举"(enum16{"读取数据", "写入数据", "读取写入DATABASE", "读取参数"}."写入数据" ("枚举")) -> ()
        n197 = Insert Into Array(array=u16[] [] ("values"), index=0 ("索引"), new element=w328) -> (w327:u16[])
        n198 = Bundle By Name(cluster=cluster{"starting address":u16, "values":u16[]} {"starting address"=0, "values"=[]}, "starting address"=w331, "values"=w327) -> (w333:cluster{"starting address":u16, "values":u16[]})
        n199 = Enqueue Element(queue=w332, element=w333) -> ()  [unwired: 2 in, 3 out]
      }
      event "启动": Mouse Down {
        n200 = event-data() -> ()  [unwired: 1 in, 8 out]
        n201 = call "启动测量模式选择对话框.vi"() -> ("启动选择 3"=w369:u16)  [unwired: 11 in]
        "启动选择 3" <- w369
        n202 = case shown="7, 默认" w369 {
          tunnel: [u16 4608 ("address") u16 4608 ("address") u16 4608 ("address") u16 4608 ("address") u16 4608 ("address") u16 4608 ("address") u16 4608 ("address") u16 4608 ("address")] -> w365
          tunnel: [u16 1 ("address") u16 2 ("address") u16 3 ("address") u16 7 ("address") u16 6 ("address") u16 8 ("address") u16 9 ("address") u16 0 ("address")] -> w362
          frame 0 {
          }
          frame 1 {
          }
          frame 2 {
          }
          frame 3 {
          }
          frame 4 {
          }
          frame 5 {
          }
          frame 6 {
          }
          frame 7, Default {
          }
        }
        n203 = local write "枚举"(enum16{"读取数据", "写入数据", "读取写入DATABASE", "读取参数"}."写入数据" ("枚举")) -> ()
        n204 = Insert Into Array(array=u16[] [] ("values"), index=0 ("索引"), new element=w362) -> (w361:u16[])
        n205 = Bundle By Name(cluster=cluster{"starting address":u16, "values":u16[]} {"starting address"=0, "values"=[]}, "starting address"=w365, "values"=w361) -> (w367:cluster{"starting address":u16, "values":u16[]})
        n206 = Enqueue Element(queue=w366, element=w367) -> ()  [unwired: 2 in, 3 out]
      }
      event "停止": Value Change {
        n207 = event-data() -> ()  [unwired: 1 in, 6 out]
        n208 = local write "枚举"(enum16{"读取数据", "写入数据", "读取写入DATABASE", "读取参数"}."写入数据" ("枚举")) -> ()
        n209 = Bundle By Name(cluster=cluster{"starting address":u16, "values":u16[]} {"starting address"=0, "values"=[]}, "starting address"=u16 4608, "values"=u16[] [11]) -> (w389:cluster{"starting address":u16, "values":u16[]})
        n210 = Enqueue Element(queue=w387, element=w389) -> ()  [unwired: 2 in, 3 out]
      }
      event "参数配置": Value Change {
        n211 = event-data() -> ()  [unwired: 1 in, 6 out]
        n212 = property on="窗格" class="Pane"("Origin"=T6 {"Horizontal"=0, "Vertical"=610} ("原点")) -> ()  [unwired: 2 in, 2 out]
        n213 = Bundle By Name(cluster=T5 {"starting address"=0, "number of holding registers"=0}, "starting address"=u16 4240, "number of holding registers"=u16 16) -> (w400:T5)
        n214 = local write "枚举"(enum16{"读取数据", "写入数据", "读取写入DATABASE", "读取参数"}."读取参数" ("枚举")) -> ()
        n215 = Flush Queue(queue=w393, error in (no error)=w392) -> (queue out=w396:refnum<queue>, error out=w395:errorcluster)  [unwired: 1 out]
        n216 = Enqueue Element(queue=w396, element=w400, error in (no error)=w395) -> ()  [unwired: 1 in, 3 out]
      }
      event "关闭": Value Change {
        n217 = event-data() -> ()  [unwired: 1 in, 6 out]
        n218 = property on="窗格" class="Pane"("Origin"=T6 {"Horizontal"=0, "Vertical"=0} ("原点")) -> ()  [unwired: 2 in, 2 out]
      }
      event Timeout; Application Instance Close {
        n219 = event-data() -> ()  [unwired: 1 in, 3 out]
        n220 = call-dynamic "Close Session.vi"("error in (no error)"=w403, "MB_Serial session"=w404) -> ()  [unwired: 9 in, 1 out]
      }
      event "时间校准": Value Change {
        n221 = event-data() -> ()  [unwired: 1 in, 6 out]
        n222 = flat-sequence {
          tunnel: w405 -> [w410]
          frame #0 {
            n223 = Get Date/Time In Seconds() -> (seconds since 1Jan1904=w415:timestamp)
            n224 = Build Array(w415) -> (w414:timestamp[])
            n225 = call "DateToHex.vi"("DATE"=w414) -> ("数组"=w408:u16[])  [unwired: 10 in]
            n226 = Insert Into Array(array=u16[] [1] ("values"), index=1 ("索引"), new element=w408) -> (w406:u16[])
            n227 = Bundle By Name(cluster=cluster{"starting address":u16, "values":u16[]} {"starting address"=0, "values"=[]}, "starting address"=u16 4612, "values"=w406) -> (w411:cluster{"starting address":u16, "values":u16[]})
            n228 = Enqueue Element(queue=w410, element=w411) -> ()  [unwired: 2 in, 3 out]
          }
          frame #1 {
            n229 = local write "枚举"(enum16{"读取数据", "写入数据", "读取写入DATABASE", "读取参数"}."写入数据" ("枚举")) -> ()
          }
        }
      }
      event "故障清除": Value Change {
        n230 = event-data() -> ()  [unwired: 1 in, 6 out]
        n231 = local write "枚举"(enum16{"读取数据", "写入数据", "读取写入DATABASE", "读取参数"}."写入数据" ("枚举")) -> ()
        n232 = Bundle By Name(cluster=cluster{"starting address":u16, "values":u16[]} {"starting address"=0, "values"=[]}, "starting address"=u16 4611, "values"=u16[] [1]) -> (w420:cluster{"starting address":u16, "values":u16[]})
        n233 = Enqueue Element(queue=w419, element=w420) -> ()  [unwired: 2 in, 3 out]
      }
      event "定时启动": Mouse Down {
        n234 = event-data() -> ()  [unwired: 1 in, 8 out]
        n235 = call "COD定时启动对话框.vi"() -> ("设置值"=→"设置值":dbl, "确定输出"=w423:bool)  [unwired: 10 in]
        n236 = local write "定时启动"(w423) -> ()
      }
    }
  }
  n237 = while {
    tunnel: w20 -> [w489]
    tunnel: w19 -> [w488]
    tunnel: w8 -> [w483]
    tunnel: w7 -> [w482]
    i -> [w484]
    stop <- FALSE stop-if-true
    n238 = Wait (ms)(milliseconds to wait=u32 1000 ("等待时间（毫秒）")) -> ()  [unwired: 1 out]
    n239 = Multiply(x="浓度 2", y=100.0) -> (x*y=w453:dbl)
    n240 = Bundle By Name(cluster=T5 {"starting address"=4224, "number of holding registers"=16}, "starting address"=u16 4224, "number of holding registers"=u16 50) -> (w547:T5)
    n241 = property on="启动选择 3" class="Ring (严格)"() -> ("RingText.Text"=w425:string)  [unwired: 2 in, 2 out]
    n242 = Multiply(x="温度", y=10.0) -> (x*y=w456:dbl)
    n243 = local write "温度 2"(w456) -> ()
    n244 = Multiply(x="修正系数 2", y=100.0) -> (x*y=w450:dbl)
    n245 = global write "COD测量模式全局.vi" "测量模式"(w425) -> ()
    n246 = local read "Registers"() -> (w541:u16[])
    n247 = Enqueue Element(queue=w489, element=w547, error in (no error)=w488) -> ()  [unwired: 1 in, 3 out]
    n248 = local write "浓度"(w453) -> ()
    n249 = Index Array(array=w541, index #1=0 ("索引"), index #4=3 ("索引"), index #14=13 ("索引"), index #15=14 ("索引"), index #32=31 ("索引")) -> (element #1=w447:u16, element #2=w446:u16, element #3=w445:u16, element #4=w511:u16, element #5=→"模式（受控）":u16, element #6=→"进样管":u16, element #7=→"高锰酸钾":u16, element #8=→"草酸钠":u16, element #9=→"硫酸":u16, element #10=→"ORP显示":u16, element #11=w518:u16, element #12=w520:u16, element #13=w533:u16, element #14=w537:u16, element #15=w491:u16, element #16=w444:u16, element #33=→"分":u16, element #34=→"秒":u16)  [unwired: 29 in, 16 out]
    "多列列表框" <- w444
    n250 = local write "修正系数"(w450) -> ()
    n251 = global write "运行时序全局变量.vi" "多列列表框"(w444) -> ()
    n252 = Divide(x=w537, y=u16 1000) -> (x/y=→"零点滴定值":dbl)
    n253 = Divide(x=w491, y=u16 1000) -> (x/y=→"标度滴定值":dbl)
    n254 = feedback #1(w444) -> (w463:u16)
    n255 = feedback-in #1(w444) -> ()
    n256 = Build Array(w447, w446, w445) -> (w448:u16[])
    n257 = Equal?(x=w520, y=u16 1) -> (x = y?=→"排液标记":bool)
    n258 = Equal?(x=w511, y=u16 0) -> (x = y?=→"待机":bool)
    n259 = Equal?(x=w511, y=u16 7) -> (x = y?=→"质控样测量":bool)
    n260 = Equal?(x=w511, y=u16 1) -> (x = y?=→"水样测量":bool)
    n261 = Equal?(x=w444, y=u16 5) -> (x = y?=w487:bool)
    n262 = Equal?(x=w511, y=u16 9) -> (x = y?=→"校标标记":bool)
    n263 = Equal?(x=w511, y=u16 6) -> (x = y?=→"平行样测量":bool)
    n264 = Equal?(x=w511, y=u16 2) -> (x = y?=→"标样核查标记":bool)
    n265 = Equal?(x=w511, y=u16 8) -> (x = y?=→"校零标记":bool)
    n266 = Equal?(x=w533, y=u16 1) -> (x = y?=w480:bool)
    "ORP故障" <- w480
    n267 = Equal?(x=w533, y=u16 2) -> (x = y?=w479:bool)
    "温控器故障" <- w479
    n268 = Equal?(x=w533, y=u16 3) -> (x = y?=w478:bool)
    "加热故障" <- w478
    n269 = Equal?(x=w533, y=u16 4) -> (x = y?=w477:bool)
    "高锰酸钾报警" <- w477
    n270 = Equal?(x=w533, y=u16 5) -> (x = y?=w476:bool)
    "草酸钠报警" <- w476
    n271 = Equal?(x=w533, y=u16 6) -> (x = y?=w475:bool)
    "测量错误" <- w475
    n272 = Equal?(x=w533, y=u16 8) -> (x = y?=w474:bool)
    "校零错误" <- w474
    n273 = Equal?(x=w533, y=u16 7) -> (x = y?=w473:bool)
    "校标错误" <- w473
    n274 = Equal?(x=w533, y=u16 9) -> (x = y?=w472:bool)
    "进水样超量程" <- w472
    n275 = Divide(x=w518, y=u16 10) -> (x/y=→"温度":dbl)
    n276 = Equal?(x=w511, y=u16 10) -> (x = y?=→"加标回收测量":bool)
    n277 = Equal?(x=w533, y=u16 10) -> (x = y?=w471:bool)
    "排液故障" <- w471
    n278 = Compound Arithmetic op=OR ("复合运算")(w480, w479, w478, w477, w476, w475, w473, w474, w472, w471) -> (→"故障标记":bool)
    n279 = Not Equal?(x=w444, y=w463) -> (x != y?=w462:bool)
    n280 = call <vilib>:"Boolean Crossing PtByPt.vi"("direction"=enum16{"either", "false-true", "true-false"}."false-true", "input"=w487) -> ("crossing"=w485:bool)  [unwired: 1 in]
    n281 = Bundle By Name(cluster=T2 {"ORP故障"=FALSE, "温控器故障"=FALSE, "加热故障"=FALSE, "高锰酸钾报警"=FALSE, "草酸钠报警"=FALSE, "测量错误"=FALSE, "校零错误"=FALSE, "校标错误"=FALSE, " 进水样超量程"=FALSE, "排液阀故障"=FALSE} ("报警簇"), "ORP故障"=w480, "温控器故障"=w479, "加热故障"=w478, "高锰酸钾报警"=w477, "草酸钠报警"=w476, "测量错误"=w475, "校零错误"=w474, "校标错误"=w473, "进水样超量程"=w472, "排液阀故障"=w471) -> (w464:T2)
    "报警簇" <- w464
    n282 = call "HexToDate.vi"("数组"=w448) -> ("DATE"=w442:timestamp[])  [unwired: 10 in]
    n283 = case shown="真" w485 {
      tunnel: w483 -> [_ w585]
      tunnel: w482 -> [_ w580]
      frame False {
      }
      frame True {
        n284 = Bundle By Name(cluster=T5 {"starting address"=0, "number of holding registers"=0}, "starting address"=u16 4101, "number of holding registers"=u16 10) -> (w584:T5)
        n285 = Enqueue Element(queue=w585, element=w584, error in (no error)=w580) -> ()  [unwired: 1 in, 3 out]
        n286 = local write "枚举"(enum16{"读取数据", "写入数据", "读取写入DATABASE", "读取参数"}."读取写入DATABASE" ("枚举")) -> ()
      }
    }
    n287 = case shown="真" w462 {
      tunnel: w444 -> [_ w563]
      frame False {
      }
      frame True {
        n288 = property on="多列列表框" class="MCListbox (严格)"() -> ("ItemNames"=w557:string[][])  [unwired: 2 in, 2 out]
        n289 = Index Array(array=w557, index (row)=w563) -> (element=w554:string[])  [unwired: 1 in]
        n290 = Index Array(array=w554, index=0 ("索引")) -> (element=w552:string)
        n291 = Array To Spreadsheet String(delimiter (Tab)="-" ("分隔符(Tab)"), array=w554, 3:"" ("格式字符串")) -> ()  [unwired: 1 out]
        n292 = Get Date/Time In Seconds() -> (seconds since 1Jan1904=w561:timestamp)
        n293 = Bundle(cluster="data in", "时间标识"=w561, "参数"="CODMn" ("table输入"), "日志信息"=w552, "流程参数"="" ("table输入")) -> (w558:T1)
        n294 = call "流程日志字段定义.vi"("table输入"="操作日志", "data in"=w558) -> ("table输出"=w566:string, "columns"=w567:string[], "data out"=w568:T9)  [unwired: 7 in]
        n295 = call "插入数据.vi"("data"=w568, "columns"=w567, "database"="database3.mdb", "table"=w566) -> ()  [unwired: 7 in, 1 out]
      }
    }
    n296 = Index Array(array=w442) -> (element=→"仪器时间":timestamp)  [unwired: 1 in]
    n297 = Get Date/Time In Seconds() -> (seconds since 1Jan1904=w441:timestamp)
    "系统时间" <- w441
    n298 = Build Array(w441) -> (w440:timestamp[])
    n299 = call "DateToHex.vi"("DATE"=w440) -> ("数组"=w439:u16[])  [unwired: 10 in]
    n300 = call "DateToHex.vi"("DATE"=w442) -> ("数组"=w434:u16[])  [unwired: 10 in]
    n301 = Index Array(array=w434, index=2 ("索引")) -> (element=w436:u16)
    n302 = Index Array(array=w439, index=2 ("索引")) -> (element=w437:u16)
    n303 = Split Number(x=w436) -> (hi(x)=w430:u8)  [unwired: 1 out]
    n304 = call "CODMn报警信息.vi"("报警簇"=w464) -> ("CODMN报警信息"=w465:string)  [unwired: 10 in]
    n305 = Split Number(x=w437) -> (hi(x)=w433:u8)  [unwired: 1 out]
    n306 = To Byte Integer(number=w430) -> (8bit integer=w429:i8)
    n307 = To Byte Integer(number=w433) -> (8bit integer=w432:i8)
    n308 = Subtract(x=w429, y=w432) -> (x-y=w431:i8)
    n309 = feedback #2(w465) -> (w466:string)
    n310 = feedback-in #2(w465) -> ()
    n311 = Not Equal?(x=w465, y="") -> (x != y?=w470:bool)
    n312 = Absolute Value(x=w431) -> (abs(x)=w428:i8)
    n313 = Greater Or Equal?(x=w428, y=i8 5) -> (x >= y?=w426:bool)
    n314 = Not Equal?(x=w465, y=w466) -> (x != y?=w467:bool)
    n315 = case shown="真" w426 {
      tunnel: w426 -> [_ w548]
      frame False {
      }
      frame True {
        n316 = flat-sequence {
          tunnel: w548 -> [_]
          frame #0 {
            n317 = property on="时间校准" class="Bool (严格)"("Val(Sgnl)"=TRUE ("时间校准")) -> ()  [unwired: 2 in, 2 out]
          }
          frame #1 {
            n318 = Wait (ms)(milliseconds to wait=u32 300 ("等待时间（毫秒）")) -> ()  [unwired: 1 out]
          }
          frame #2 {
            n319 = property on="时间校准" class="Bool (严格)"("Val(Sgnl)"=FALSE ("时间校准")) -> ()  [unwired: 2 in, 2 out]
          }
        }
      }
    }
    n320 = And(x=w467, y=w470) -> (x .and. y?=w468:bool)
    n321 = case shown="真" w468 {
      tunnel: w465 -> [_ w569]
      frame False {
      }
      frame True {
        n322 = Get Date/Time In Seconds() -> (seconds since 1Jan1904=w571:timestamp)
        n323 = Bundle By Name(cluster=T8 {"时间标识"=timestamp(0 s since 1904-01-01), "设备"="", "日志信息"=""} ("data in"), "时间标识"=w571, "设备"="CODMn", "日志信息"=w569) -> (w572:T8)
        n324 = call "报警信息字段定义.vi"("table输入"="报警信息", "data in"=w572) -> ("table输出"=w576:string, "columns"=w577:string[], "data out"=w578:T8)  [unwired: 7 in]
        n325 = call "插入数据.vi"("data"=w578, "columns"=w577, "database"="database3.mdb", "table"=w576) -> ()  [unwired: 7 in, 1 out]
      }
    }
    "循环次数" <- w484
  }
  n326 = call-dynamic "Close Session.vi"("error in (no error)"=w18, "MB_Serial session"=w17) -> ()  [unwired: 9 in, 1 out]
